vi "GetReady.vi"(4 "error in (no error)":errorcluster, 6 "Timeout, (10000 ms)":i32=10000, 7 "connection ID":refnum<k5>) -> (0 "error out":errorcluster)   [LabVIEW 2011]
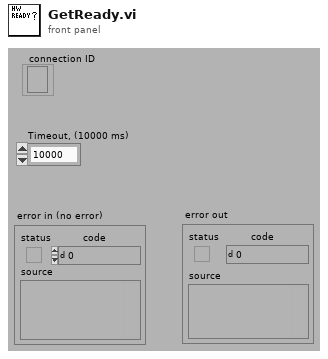
[diagram p1: front panel]
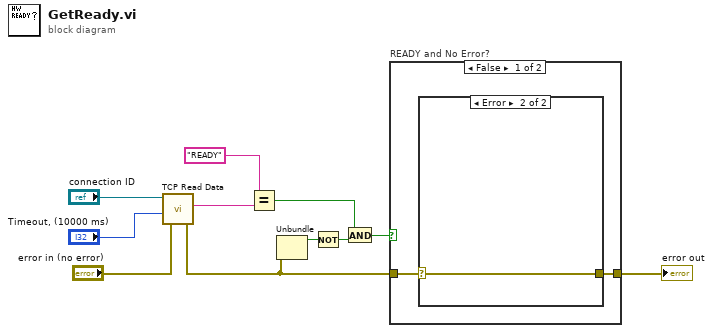
[diagram p0: block diagram]
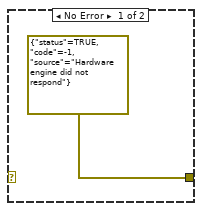
[diagram p2: hidden frame]
diagram:
  n1 = call "TCP Read Data.vi"("error in (no error)"="error in (no error)", "Timeout (25000 ms)"="Timeout, (10000 ms)", "connection ID"="connection ID") -> ("error out"=w2:errorcluster, "Flat Data"=w1:string)  [unwired: 3 out]
  n2 = Equal?(x="READY", y=w1) -> (x = y?=w9:bool)
  n3 = Unbundle(w2) -> ("status"=w10:bool)  [unwired: 2 out]
  n4 = Not(x=w10) -> (.not. x?=w7:bool)
  n5 = And(x=w9, y=w7) -> (x .and. y?=w8:bool)
  n6 = case "READY and No Error?" shown="False" w8 {
    tunnel: w2 -> [w12 w16]
    tunnel: [w13 w16] -> w11
    frame False {
      n7 = case shown="Error" w12 {
        selector: w12 -> [_ w15]
        tunnel: [errorcluster {"status"=TRUE, "code"=-1, "source"="Hardware engine did not respond"} ("error in (no error)") w15] -> w13
        frame No Error {
        }
        frame Error {
        }
      }
    }
    frame True {
    }
  }
  "error out" <- w11
